vi "AddLoggingGlobals.vi"(5 "Sequence Context":refnum<k7>) -> (0 "error out":errorcluster)   [LabVIEW 2013, in "Logger.lvlib"]
uses:
  Logger.lvlib
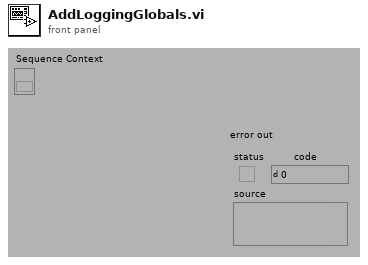
[diagram p1: front panel]
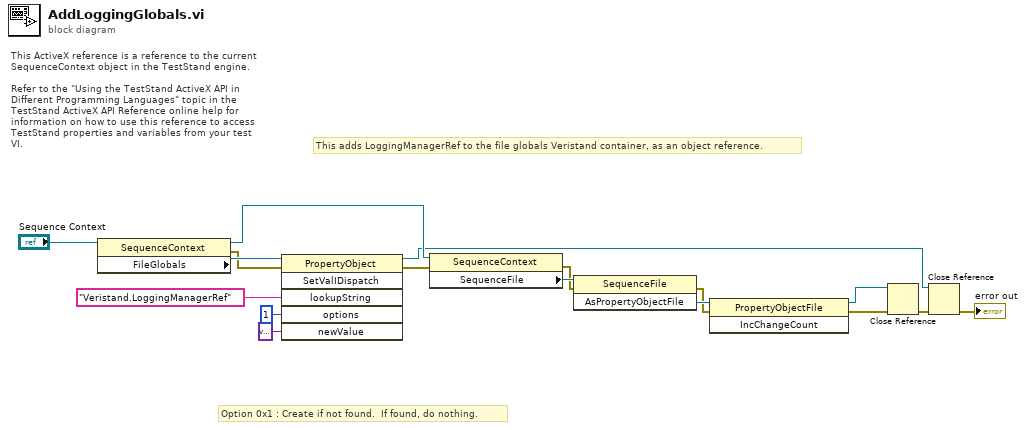
[diagram p0: block diagram]
diagram:
  # "This adds LoggingManagerRef to the file globals Veristand container, as an object reference."
  # "Option 0x1 : Create if not found.  If found, do nothing."
  # "This ActiveX reference is a reference to the current\nSequenceContext object in the TestStand engine.\n\nRefer to the \"Using the TestStand ActiveX API in\nDifferent Programming Languages\" topic in the \nTestStand ActiveX API Reference online help for\ninformation on how to use this reference to access\nTestStand properties and variables from your test VI."
  n1 = property class="SequenceContext"(reference="Sequence Context") -> (reference out=w16:refnum<k7>, error out=w8:errorcluster, "FileGlobals"=w17:refnum<k7>)  [unwired: 1 in]
  n2 = invoke class="PropertyObject" method="SetValIDispatch"(reference=w17, error in=w8, "lookupString"="Veristand.LoggingManagerRef", "options"=1, "newValue"=variant) -> (reference out=w2:refnum<k7>, error out=w1:errorcluster)  [unwired: 1 in, 4 out]
  n3 = property class="SequenceContext"(reference=w16, error in=w1) -> (error out=w14:errorcluster, "SequenceFile"=w15:refnum<k7>)  [unwired: 1 out]
  n4 = invoke class="SequenceFile" method="AsPropertyObjectFile"(reference=w15, error in=w14) -> (error out=w12:errorcluster, "AsPropertyObjectFile"=w13:refnum<k7>)  [unwired: 1 in, 1 out]
  n5 = invoke class="PropertyObjectFile" method="IncChangeCount"(reference=w13, error in=w12) -> (reference out=w10:refnum<k7>, error out=w11:errorcluster)  [unwired: 1 in, 1 out]
  n6 = Close Reference(reference=w10, error in (no error)=w11) -> (error out=w9:errorcluster)
  n7 = Close Reference(reference=w2, error in (no error)=w9) -> (error out=→"error out":errorcluster)
